vi "Sub_Build_MQTT_String.vi"(8 "error in (no error)":errorcluster, 10 "String to be encoded":string="MQIsdp") -> (0 "error out":errorcluster, 2 "UTF8 Byte Array":u8[](array[numeric]) format="%x")   [LabVIEW 2013, in "IOTFoundation.lvlib"]
uses:
  IOTFoundation.lvlib
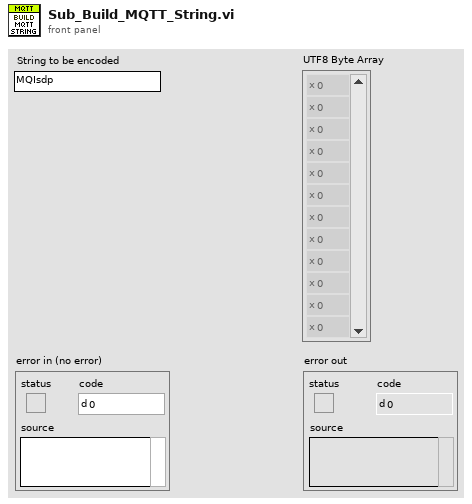
[diagram p1: front panel]
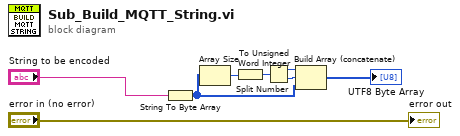
[diagram p0: block diagram]
diagram:
  n1 = String To Byte Array(string="String to be encoded") -> (unsigned byte array=w8:u8[])
  n2 = Array Size(array=w8) -> (size(s)=w7:i32)
  n3 = To Unsigned Word Integer(number=w7) -> (unsigned 16bit integer=w3:u16)
  n4 = Split Number(x=w3) -> (hi(x)=w5:u8, lo(x)=w6:u8)
  n5 = Build Array (concatenate)(w5, w6, w8) -> (→"UTF8 Byte Array":u8[])
  "error out" <- "error in (no error)"
